vi "PDF Standard Kopf Gas Flasche Komponenten.vi"(10 "Gasnummer Index":i32, 11 "Komponenten":T1[](array[typedef]) {"Konzentration IST" format="%#.4f"; "Genauigkeit" format="%#.1f"}) -> (1 "Konzentration IST":string, 2 "Gasauswahl":string, 3 "Genauigkeit":string)   [LabVIEW 2020, in "PDF Interface.lvlib"]
uses:
  Seiten/System Einstellungen V2/Gasflaschenkomponente.ctl
  PDF Interface.lvlib
  Seiten/System Einstellungen V2/System Einstellungen V2.lvlib
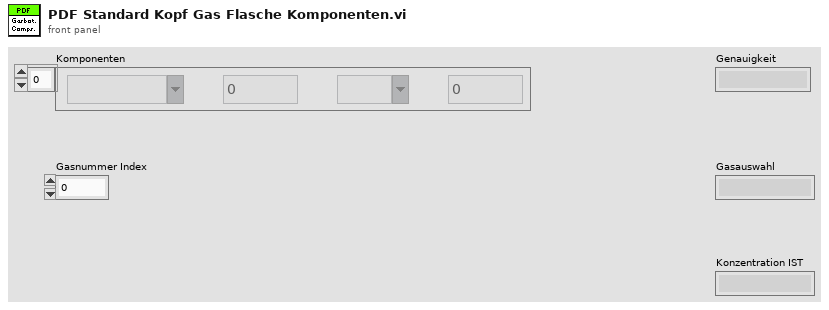
[diagram p1: front panel]
types:
  T1 = typedef "System Einstellungen V2.lvlib/Gasflaschenkomponente.ctl" = cluster{"Gasauswahl":string, "Konzentration IST":dbl, "Einheit":string, "Genauigkeit":dbl}
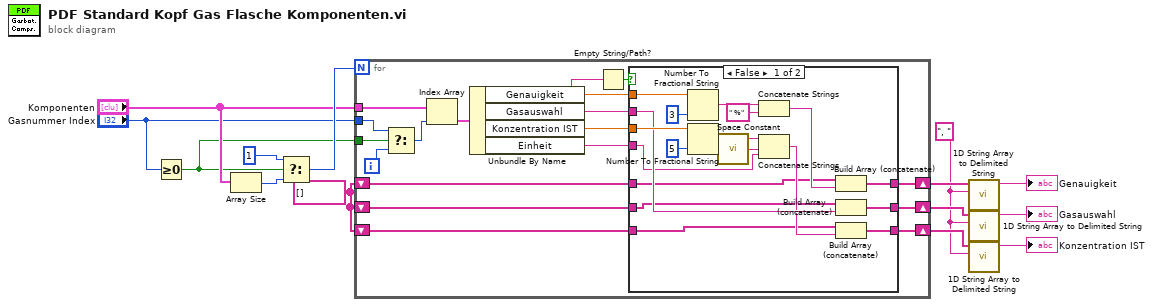
[diagram p0: block diagram]
diagram:
  w2 = ", "
  w8 = string[] []
  n1 = Greater Or Equal To 0?(x="Gasnummer Index") -> (x >= 0?=w9:bool)
  n2 = Array Size(array="Komponenten") -> (size(s)=w12:i32)
  n3 = Select(t=1 ("Gasnummer Index"), s=w9, f=w12) -> (s? t:f=w14:i32)
  n4 = for {
    N: w14 -> [_]
    tunnel: "Komponenten" -> [w31]
    tunnel: "Gasnummer Index" -> [w30]
    tunnel: w9 -> [w29]
    shift-right: [w20] -> w7
    shift-left: w8 -> [w17]
    shift-right: [w19] -> w4
    shift-left: w8 -> [w16]
    shift-right: [w18] -> w3
    shift-left: w8 -> [w15]
    i -> [w28]
    n5 = Select(t=w30, s=w29, f=w28) -> (s? t:f=w27:i32)
    n6 = Index Array(array=w31, index=w27) -> (element=w26:T1)
    n7 = Unbundle By Name(w26) -> ("Genauigkeit"=w24:dbl, "Gasauswahl"=w23:string, "Konzentration IST"=w22:dbl, "Einheit"=w21:string)
    n8 = Empty String/Path?(string/path=w23) -> (empty?=w25:bool)
    n9 = case shown="False" w25 {
      tunnel: w24 -> [w46 _]
      tunnel: w23 -> [w40 _]
      tunnel: w22 -> [w42 _]
      tunnel: w21 -> [w38 _]
      tunnel: [w37 w52] -> w20
      tunnel: [w36 w51] -> w19
      tunnel: [w35 w50] -> w18
      tunnel: w17 -> [w34 w52]
      tunnel: w16 -> [w33 w51]
      tunnel: w15 -> [w32 w50]
      frame False {
        n10 = Number To Fractional String(number=w46, precision (6)=i16 3 ("Genauigkeit (6)")) -> (F-format string=w48:string)  [unwired: 2 in]
        n11 = Number To Fractional String(number=w42, precision (6)=i16 5 ("Genauigkeit (6)")) -> (F-format string=w44:string)  [unwired: 2 in]
        n12 = call <vilib>:"Space Constant.vi"() -> ("String"=w43:string)
        n13 = Concatenate Strings(w48, " %" ("String")) -> (w41:string)
        n14 = Concatenate Strings(w44, w43, w38) -> (w39:string)
        n15 = Build Array (concatenate)(w34, w41) -> (w37:string[])
        n16 = Build Array (concatenate)(w33, w40) -> (w36:string[])
        n17 = Build Array (concatenate)(w32, w39) -> (w35:string[])
      }
      frame True {
      }
    }
  }
  n18 = call <vilib>:"1D String Array to Delimited String.vi"("delimiter"=w2, "string array"=w7) -> ("delimited string"=→"Genauigkeit":string)  [unwired: 9 in]
  n19 = call <vilib>:"1D String Array to Delimited String.vi"("delimiter"=w2, "string array"=w4) -> ("delimited string"=→"Gasauswahl":string)  [unwired: 9 in]
  n20 = call <vilib>:"1D String Array to Delimited String.vi"("delimiter"=w2, "string array"=w3) -> ("delimited string"=→"Konzentration IST":string)  [unwired: 9 in]
